vi "Transmit.vi"(8 "error in (no error)":errorcluster, 9 "Frame":string, 10 "Data in":refnum<class "XNET Data.lvclass">, 11 "CAN in":refnum<class "XNET_BS120x.lvclass">) -> (0 "error out":errorcluster, 3 "CAN out":refnum<class "XNET_BS120x.lvclass">)   [LabVIEW 2021, in "BS120x Driver.lvlib" / "XNET_BS120x.lvclass"]
uses:
  XNET_BS120x.lvclass
  _Private/Data Classes/XNET Data Class/XNET Data.lvclass
  _Private/Data Classes/XNET Data Class/XNET Data.lvclass/XNET Data.ctl
  XNET_BS120x.lvclass/XNET_BS120x.ctl
  _Private/Data Classes/XNET Data Class/Read XNET Array.vi
  <vilib>/xnet/xnet.llb/XNET Write (Frame CAN).vi
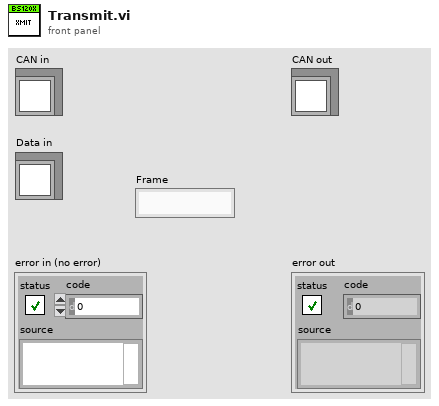
[diagram p1: front panel]
types:
  T1 = typedef "XNET Frame CAN.ctl" = cluster{"timestamp":timestamp, "payload":u8[], "identifier":u32, "type":T2, "extended?":bool, "echo?":bool}
  T2 = typedef "XNET Frame Type CAN.ctl" = u8
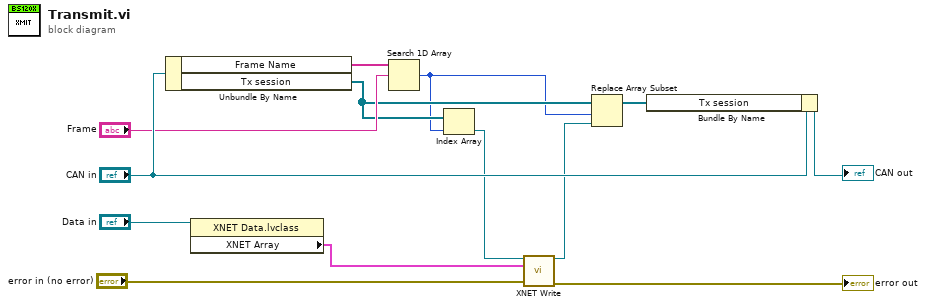
[diagram p0: block diagram]
diagram:
  n1 = Unbundle By Name("CAN in") -> ("Frame Name"=w6:string[], "Tx session"=w5:refnum<k21>[])
  n2 = property class="XNET Data.lvclass"(reference="Data in") -> ("XNET Array"=w13:T1[])  [unwired: 1 in, 2 out]
  n3 = Search 1D Array(1D array=w6, element="Frame") -> (index of element=w3:i32)  [unwired: 1 in]
  n4 = Index Array(array=w5, index=w3) -> (element=w7:refnum<k21>)
  n5 = call-poly <vilib>:"XNET Write.vi"("session in"=w7, "data"=w13, "error in (no error)"="error in (no error)") -> ("session out"=w4:refnum<k21>, "error out"=→"error out":errorcluster)  [unwired: 11 out]
  n6 = Replace Array Subset(array=w5, new element=w4, index=w3) -> (w1:refnum<k21>[])
  n7 = Bundle By Name(cluster="CAN in", "Tx session"=w1) -> (→"CAN out":refnum<class "XNET_BS120x.lvclass">)
